vi "LED Control.vi"(11 "All Robot Commands In":T5) -> ()   [LabVIEW 2016]
uses:
  Drive and Climb SS/Drive + Climb Commands 2017.ctl
  Gear Delivery SS/Gear Delivery Commands.ctl
  Conveyor and Shooter SS/Conveyor and Shooter Commands.ctl
  Ball Intake SS/Ball Intake Commands.ctl
  Global Variables/Refnum Names.vi
  Global Variables/Robot Status.vi
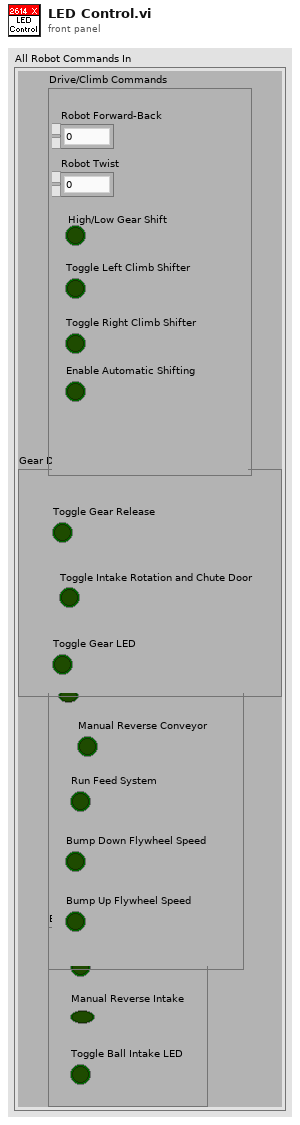
[diagram p1: front panel]
types:
  T1 = typedef "Drive + Climb Commands 2017.ctl" = cluster{"Robot Forward-Back":dbl, "Robot Twist":dbl, "High/Low Gear Shift":bool, "Toggle Left Climb Shifter":bool, "Toggle Right Climb Shifter":bool, "Enable Automatic Shifting":bool}
  T2 = typedef "Gear Delivery Commands.ctl" = cluster{"Toggle Gear Release":bool, "Toggle Intake Rotation and Chute Door":bool, "Toggle Gear LED":bool}
  T3 = typedef "Conveyor and Shooter Commands.ctl" = cluster{"Toggle Shooter":bool, "Manual Reverse Conveyor":bool, "Run Feed System":bool, "Bump Down Flywheel Speed":bool, "Bump Up Flywheel Speed":bool}
  T4 = typedef "Ball Intake Commands.ctl" = cluster{"Toggle Ball Intake":bool, "Manual Reverse Intake":bool, "Toggle Ball Intake LED":bool}
  T5 = cluster{"Drive/Climb Commands":T1, "Gear Delivery Commands":T2, "Shooter and Conveyor Commands":T3, "Ball Intake Commands":T4}
  T6 = typedef "WPI_MotorControlDeviceRef.ctl" = cluster{"DeviceStatus":errorcluster, "Type":T7, "PWM":cluster{"PWM Channel":T8, "DeadBand":T9}, "CAN":cluster{"Device Number":u8, "SetOutput VI Ref":variant, "GetOutput VI Ref":variant, "Enable VI Ref":variant, "Disable VI Ref":variant, "Data":variant}, "Invert":bool}
  T7 = typedef "WPI_MotorControlType.ctl" = enum16{"PWM", "CAN"}
  T8 = typedef "FPGA_DIOPWMChannel.ctl" = enum8{"PWM 0", "PWM 1", "PWM 2", "PWM 3", "PWM 4", "PWM 5", "PWM 6", "PWM 7", "PWM 8", "PWM 9", "PWM MXP 0", "PWM MXP 1", "PWM MXP 2", "PWM MXP 3", "PWM MXP 4", "PWM MXP 5", "PWM MXP 6", "PWM MXP 7", "PWM MXP 8", "PWM MXP 9", "Invalid"}
  T9 = typedef "WPI_PWMDeadband.ctl" = cluster{"Name":string, "maxPositivePwm":i32, "minPositivePwm":i32, "centerPwm":i32, "maxNegativePwm":i32, "minNegativePwm":i32, "angularRange":u16}
  T10 = typedef "WPI_DigitalOutputDevRef.ctl" = cluster{"DIO Channel":T11, "DevStatus":errorcluster}
  T11 = typedef "FPGA_DIOChannel.ctl" = enum8{"DIO 0", "DIO 1", "DIO 2", "DIO 3", "DIO 4", "DIO 5", "DIO 6", "DIO 7", "DIO 8", "DIO 9", "DIO MXP 0", "DIO MXP 1", "DIO MXP 2", "DIO MXP 3", "DIO MXP 4", "DIO MXP 5", "DIO MXP 6", "DIO MXP 7", "DIO MXP 8", "DIO MXP 9", "DIO MXP 10", "DIO MXP 11", "DIO MXP 12", "DIO MXP 13", "DIO MXP 14", "DIO MXP 15", "SPI Port CS1", "SPI Port CS2", "SPI Port CS3", "SPI Port MISO", "SPI Port MOSI", "Invalid"}
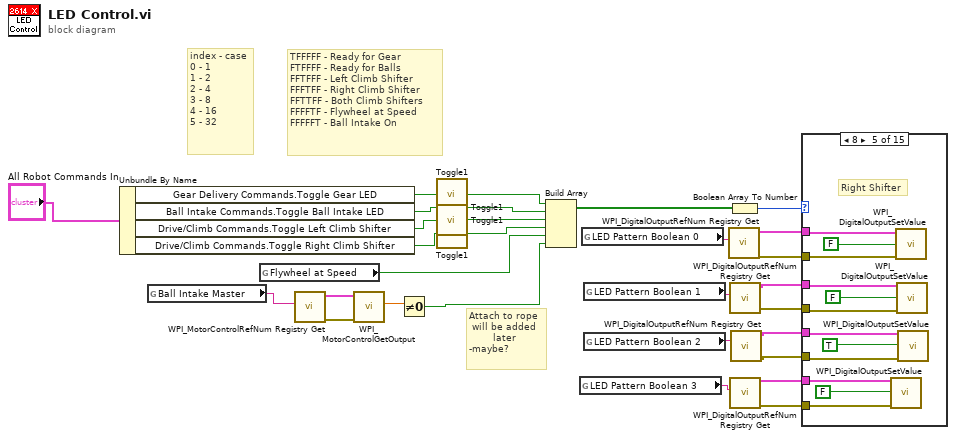
[diagram p0: block diagram]
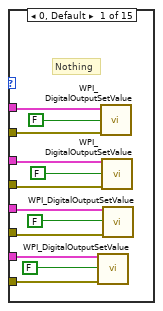
[diagram p2: hidden frame]
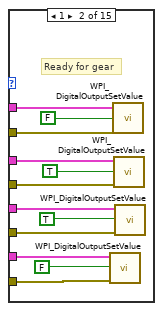
[diagram p3: hidden frame]
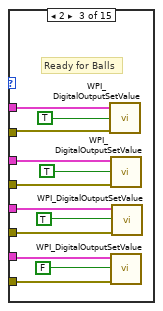
[diagram p4: hidden frame]
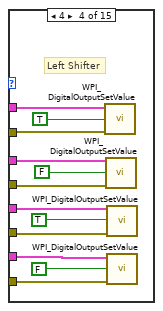
[diagram p5: hidden frame]
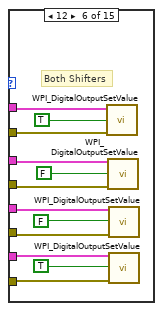
[diagram p6: hidden frame]
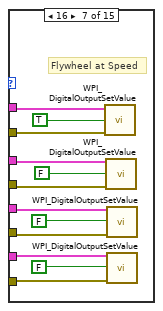
[diagram p7: hidden frame]
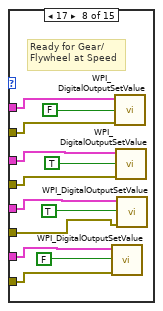
[diagram p8: hidden frame]
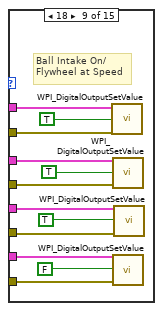
[diagram p9: hidden frame]
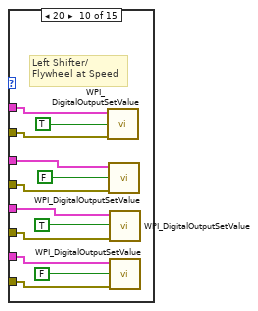
[diagram p10: hidden frame]
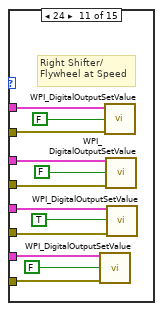
[diagram p11: hidden frame]
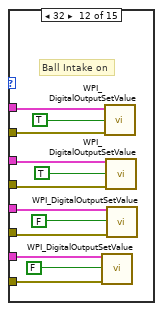
[diagram p12: hidden frame]
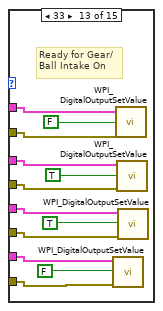
[diagram p13: hidden frame]
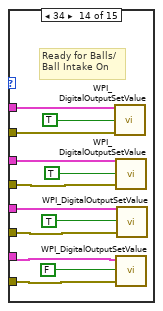
[diagram p14: hidden frame]
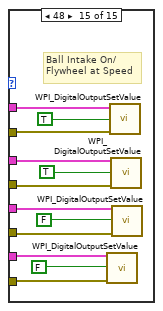
[diagram p15: hidden frame]
diagram:
  # "index - case\n0 - 1\n1 - 2\n2 - 4\n3 - 8\n4 - 16\n5 - 32"
  # "TFFFFF - Ready for Gear\nFTFFFF - Ready for Balls\nFFTFFF - Left Climb Shifter\nFFFTFF - Right Climb Shifter\nFFTTFF - Both Climb Shifters\nFFFFTF - Flywheel at Speed\nFFFFFT - Ball Intake On"
  # "Attach to rope\n will be added \n        later\n-maybe?"
  n1 = Unbundle By Name("All Robot Commands In") -> ("Gear Delivery Commands.Toggle Gear LED"=w11:bool, "Ball Intake Commands.Toggle Ball Intake LED"=w9:bool, "Drive/Climb Commands.Toggle Left Climb Shifter"=w15:bool, "Drive/Climb Commands.Toggle Right Climb Shifter"=w14:bool)
  n2 = global read "Refnum Names.vi" "Ball Intake Master"() -> (w8:string)
  n3 = global read "Robot Status.vi" "Flywheel at Speed"() -> (w4:bool)
  n4 = call <vilib>:"WPI_MotorControlRefNum Registry Get.vi"("refnum name"=w8) -> ("error out"=w7:errorcluster, "MotorControlDevRef"=w6:T6)  [unwired: 9 in]
  n5 = call <vilib>:"WPI_MotorControlGetOutput.vi"("error in"=w7, "MotorControlDevRef"=w6) -> ("Output"=w5:dbl)  [unwired: 7 in, 2 out]
  n6 = Not Equal To 0?(x=w5) -> (x != 0?=w3:bool)
  n7 = call "Toggle1.vi"("Boolean"=w11) -> ("Driver Switch 2"=w1:bool)
  n8 = call "Toggle1.vi"("Boolean"=w9) -> ("Driver Switch 2"=w10:bool)
  n9 = call "Toggle1.vi"("Boolean"=w15) -> ("Driver Switch 2"=w2:bool)
  n10 = call "Toggle1.vi"("Boolean"=w14) -> ("Driver Switch 2"=w12:bool)
  n11 = Build Array(w1, w10, w2, w12, w4, w3) -> (w22:bool[])
  n12 = global read "Refnum Names.vi" "LED Pattern Boolean 3"() -> (w13:string)
  n13 = global read "Refnum Names.vi" "LED Pattern Boolean 0"() -> (w20:string)
  n14 = global read "Refnum Names.vi" "LED Pattern Boolean 1"() -> (w18:string)
  n15 = global read "Refnum Names.vi" "LED Pattern Boolean 2"() -> (w19:string)
  n16 = call <vilib>:"WPI_DigitalOutputRefNum Registry Get.vi"("refnum name"=w20) -> ("error out"=w28:errorcluster, "DigitalOutputDevRef"=w23:T10)  [unwired: 9 in]
  n17 = Boolean Array To Number(Boolean array=w22) -> (number=w21:u32)
  n18 = call <vilib>:"WPI_DigitalOutputRefNum Registry Get.vi"("refnum name"=w18) -> ("error out"=w26:errorcluster, "DigitalOutputDevRef"=w27:T10)  [unwired: 9 in]
  n19 = call <vilib>:"WPI_DigitalOutputRefNum Registry Get.vi"("refnum name"=w13) -> ("error out"=w16:errorcluster, "DigitalOutputDevRef"=w17:T10)  [unwired: 9 in]
  n20 = call <vilib>:"WPI_DigitalOutputRefNum Registry Get.vi"("refnum name"=w19) -> ("error out"=w24:errorcluster, "DigitalOutputDevRef"=w25:T10)  [unwired: 9 in]
  n21 = case shown="8" w21 {
    tunnel: w23 -> [w38 w50 w62 w74 w86 w99 w110 w121 w133 w145 w158 w170 w181 w193 w205]
    tunnel: w28 -> [w37 w49 w61 w73 w85 w98 w109 w120 w132 w144 w157 w169 w180 w192 w204]
    tunnel: w27 -> [w36 w48 w60 w72 w84 w97 w108 w119 w131 w143 w156 w168 w179 w191 w203]
    tunnel: w26 -> [w35 w47 w59 w71 w83 w96 w107 w118 w130 w142 w155 w167 w178 w190 w202]
    tunnel: w25 -> [w34 w46 w58 w70 w82 w95 w106 w117 w129 w141 w154 w166 w177 w189 w201]
    tunnel: w24 -> [w33 w45 w57 w69 w81 w94 w105 w116 w128 w140 w153 w165 w176 w188 w200]
    tunnel: w17 -> [w32 w43 w55 w67 w79 w93 w104 w115 w127 w139 w152 w163 w175 w187 w199]
    tunnel: w16 -> [w30 w42 w54 w66 w78 w92 w103 w114 w126 w138 w151 w162 w174 w186 w198]
    frame 0, Default {
      # "Nothing"
      n22 = call <vilib>:"WPI_DigitalOutputSetValue.vi"("error in (no error)"=w30, "Value"=FALSE, "DigitalOutputDevRef"=w32) -> ()  [unwired: 7 in, 2 out]
      n23 = call <vilib>:"WPI_DigitalOutputSetValue.vi"("error in (no error)"=w37, "Value"=FALSE, "DigitalOutputDevRef"=w38) -> ()  [unwired: 7 in, 2 out]
      n24 = call <vilib>:"WPI_DigitalOutputSetValue.vi"("error in (no error)"=w35, "Value"=FALSE, "DigitalOutputDevRef"=w36) -> ()  [unwired: 7 in, 2 out]
      n25 = call <vilib>:"WPI_DigitalOutputSetValue.vi"("error in (no error)"=w33, "Value"=FALSE, "DigitalOutputDevRef"=w34) -> ()  [unwired: 7 in, 2 out]
    }
    frame 1 {
      # "Ready for gear"
      n26 = call <vilib>:"WPI_DigitalOutputSetValue.vi"("error in (no error)"=w42, "Value"=FALSE, "DigitalOutputDevRef"=w43) -> ()  [unwired: 7 in, 2 out]
      n27 = call <vilib>:"WPI_DigitalOutputSetValue.vi"("error in (no error)"=w49, "Value"=FALSE, "DigitalOutputDevRef"=w50) -> ()  [unwired: 7 in, 2 out]
      n28 = call <vilib>:"WPI_DigitalOutputSetValue.vi"("error in (no error)"=w47, "Value"=TRUE, "DigitalOutputDevRef"=w48) -> ()  [unwired: 7 in, 2 out]
      n29 = call <vilib>:"WPI_DigitalOutputSetValue.vi"("error in (no error)"=w45, "Value"=TRUE, "DigitalOutputDevRef"=w46) -> ()  [unwired: 7 in, 2 out]
    }
    frame 2 {
      # "Ready for Balls"
      n30 = call <vilib>:"WPI_DigitalOutputSetValue.vi"("error in (no error)"=w61, "Value"=TRUE, "DigitalOutputDevRef"=w62) -> ()  [unwired: 7 in, 2 out]
      n31 = call <vilib>:"WPI_DigitalOutputSetValue.vi"("error in (no error)"=w59, "Value"=TRUE, "DigitalOutputDevRef"=w60) -> ()  [unwired: 7 in, 2 out]
      n32 = call <vilib>:"WPI_DigitalOutputSetValue.vi"("error in (no error)"=w54, "Value"=FALSE, "DigitalOutputDevRef"=w55) -> ()  [unwired: 7 in, 2 out]
      n33 = call <vilib>:"WPI_DigitalOutputSetValue.vi"("error in (no error)"=w57, "Value"=TRUE, "DigitalOutputDevRef"=w58) -> ()  [unwired: 7 in, 2 out]
    }
    frame 4 {
      # "Left Shifter"
      n34 = call <vilib>:"WPI_DigitalOutputSetValue.vi"("error in (no error)"=w73, "Value"=TRUE, "DigitalOutputDevRef"=w74) -> ()  [unwired: 7 in, 2 out]
      n35 = call <vilib>:"WPI_DigitalOutputSetValue.vi"("error in (no error)"=w71, "Value"=FALSE, "DigitalOutputDevRef"=w72) -> ()  [unwired: 7 in, 2 out]
      n36 = call <vilib>:"WPI_DigitalOutputSetValue.vi"("error in (no error)"=w69, "Value"=TRUE, "DigitalOutputDevRef"=w70) -> ()  [unwired: 7 in, 2 out]
      n37 = call <vilib>:"WPI_DigitalOutputSetValue.vi"("error in (no error)"=w66, "Value"=FALSE, "DigitalOutputDevRef"=w67) -> ()  [unwired: 7 in, 2 out]
    }
    frame 8 {
      # "Right Shifter"
      n38 = call <vilib>:"WPI_DigitalOutputSetValue.vi"("error in (no error)"=w78, "Value"=FALSE, "DigitalOutputDevRef"=w79) -> ()  [unwired: 7 in, 2 out]
      n39 = call <vilib>:"WPI_DigitalOutputSetValue.vi"("error in (no error)"=w85, "Value"=FALSE, "DigitalOutputDevRef"=w86) -> ()  [unwired: 7 in, 2 out]
      n40 = call <vilib>:"WPI_DigitalOutputSetValue.vi"("error in (no error)"=w83, "Value"=FALSE, "DigitalOutputDevRef"=w84) -> ()  [unwired: 7 in, 2 out]
      n41 = call <vilib>:"WPI_DigitalOutputSetValue.vi"("error in (no error)"=w81, "Value"=TRUE, "DigitalOutputDevRef"=w82) -> ()  [unwired: 7 in, 2 out]
    }
    frame 12 {
      # "Both Shifters"
      n42 = call <vilib>:"WPI_DigitalOutputSetValue.vi"("error in (no error)"=w98, "Value"=TRUE, "DigitalOutputDevRef"=w99) -> ()  [unwired: 7 in, 2 out]
      n43 = call <vilib>:"WPI_DigitalOutputSetValue.vi"("error in (no error)"=w96, "Value"=FALSE, "DigitalOutputDevRef"=w97) -> ()  [unwired: 7 in, 2 out]
      n44 = call <vilib>:"WPI_DigitalOutputSetValue.vi"("error in (no error)"=w94, "Value"=FALSE, "DigitalOutputDevRef"=w95) -> ()  [unwired: 7 in, 2 out]
      n45 = call <vilib>:"WPI_DigitalOutputSetValue.vi"("error in (no error)"=w92, "Value"=TRUE, "DigitalOutputDevRef"=w93) -> ()  [unwired: 7 in, 2 out]
    }
    frame 16 {
      # "Flywheel at Speed"
      n46 = call <vilib>:"WPI_DigitalOutputSetValue.vi"("error in (no error)"=w109, "Value"=TRUE, "DigitalOutputDevRef"=w110) -> ()  [unwired: 7 in, 2 out]
      n47 = call <vilib>:"WPI_DigitalOutputSetValue.vi"("error in (no error)"=w107, "Value"=FALSE, "DigitalOutputDevRef"=w108) -> ()  [unwired: 7 in, 2 out]
      n48 = call <vilib>:"WPI_DigitalOutputSetValue.vi"("error in (no error)"=w105, "Value"=FALSE, "DigitalOutputDevRef"=w106) -> ()  [unwired: 7 in, 2 out]
      n49 = call <vilib>:"WPI_DigitalOutputSetValue.vi"("error in (no error)"=w103, "Value"=FALSE, "DigitalOutputDevRef"=w104) -> ()  [unwired: 7 in, 2 out]
    }
    frame 17 {
      # "Ready for Gear/\nFlywheel at Speed"
      n50 = call <vilib>:"WPI_DigitalOutputSetValue.vi"("error in (no error)"=w114, "Value"=FALSE, "DigitalOutputDevRef"=w115) -> ()  [unwired: 7 in, 2 out]
      n51 = call <vilib>:"WPI_DigitalOutputSetValue.vi"("error in (no error)"=w120, "Value"=FALSE, "DigitalOutputDevRef"=w121) -> ()  [unwired: 7 in, 2 out]
      n52 = call <vilib>:"WPI_DigitalOutputSetValue.vi"("error in (no error)"=w118, "Value"=TRUE, "DigitalOutputDevRef"=w119) -> ()  [unwired: 7 in, 2 out]
      n53 = call <vilib>:"WPI_DigitalOutputSetValue.vi"("error in (no error)"=w116, "Value"=TRUE, "DigitalOutputDevRef"=w117) -> ()  [unwired: 7 in, 2 out]
    }
    frame 18 {
      # "Ball Intake On/\nFlywheel at Speed"
      n54 = call <vilib>:"WPI_DigitalOutputSetValue.vi"("error in (no error)"=w132, "Value"=TRUE, "DigitalOutputDevRef"=w133) -> ()  [unwired: 7 in, 2 out]
      n55 = call <vilib>:"WPI_DigitalOutputSetValue.vi"("error in (no error)"=w130, "Value"=TRUE, "DigitalOutputDevRef"=w131) -> ()  [unwired: 7 in, 2 out]
      n56 = call <vilib>:"WPI_DigitalOutputSetValue.vi"("error in (no error)"=w126, "Value"=FALSE, "DigitalOutputDevRef"=w127) -> ()  [unwired: 7 in, 2 out]
      n57 = call <vilib>:"WPI_DigitalOutputSetValue.vi"("error in (no error)"=w128, "Value"=TRUE, "DigitalOutputDevRef"=w129) -> ()  [unwired: 7 in, 2 out]
    }
    frame 20 {
      # "Left Shifter/\nFlywheel at Speed"
      n58 = call <vilib>:"WPI_DigitalOutputSetValue.vi"("error in (no error)"=w144, "Value"=TRUE, "DigitalOutputDevRef"=w145) -> ()  [unwired: 7 in, 2 out]
      n59 = call <vilib>:"WPI_DigitalOutputSetValue.vi"("error in (no error)"=w142, "Value"=FALSE, "DigitalOutputDevRef"=w143) -> ()  [unwired: 7 in, 2 out]
      n60 = call <vilib>:"WPI_DigitalOutputSetValue.vi"("error in (no error)"=w140, "Value"=TRUE, "DigitalOutputDevRef"=w141) -> ()  [unwired: 7 in, 2 out]
      n61 = call <vilib>:"WPI_DigitalOutputSetValue.vi"("error in (no error)"=w138, "Value"=FALSE, "DigitalOutputDevRef"=w139) -> ()  [unwired: 7 in, 2 out]
    }
    frame 24 {
      # "Right Shifter/\nFlywheel at Speed"
      n62 = call <vilib>:"WPI_DigitalOutputSetValue.vi"("error in (no error)"=w151, "Value"=FALSE, "DigitalOutputDevRef"=w152) -> ()  [unwired: 7 in, 2 out]
      n63 = call <vilib>:"WPI_DigitalOutputSetValue.vi"("error in (no error)"=w157, "Value"=FALSE, "DigitalOutputDevRef"=w158) -> ()  [unwired: 7 in, 2 out]
      n64 = call <vilib>:"WPI_DigitalOutputSetValue.vi"("error in (no error)"=w155, "Value"=FALSE, "DigitalOutputDevRef"=w156) -> ()  [unwired: 7 in, 2 out]
      n65 = call <vilib>:"WPI_DigitalOutputSetValue.vi"("error in (no error)"=w153, "Value"=TRUE, "DigitalOutputDevRef"=w154) -> ()  [unwired: 7 in, 2 out]
    }
    frame 32 {
      # "Ball Intake on"
      n66 = call <vilib>:"WPI_DigitalOutputSetValue.vi"("error in (no error)"=w162, "Value"=FALSE, "DigitalOutputDevRef"=w163) -> ()  [unwired: 7 in, 2 out]
      n67 = call <vilib>:"WPI_DigitalOutputSetValue.vi"("error in (no error)"=w169, "Value"=TRUE, "DigitalOutputDevRef"=w170) -> ()  [unwired: 7 in, 2 out]
      n68 = call <vilib>:"WPI_DigitalOutputSetValue.vi"("error in (no error)"=w167, "Value"=TRUE, "DigitalOutputDevRef"=w168) -> ()  [unwired: 7 in, 2 out]
      n69 = call <vilib>:"WPI_DigitalOutputSetValue.vi"("error in (no error)"=w165, "Value"=FALSE, "DigitalOutputDevRef"=w166) -> ()  [unwired: 7 in, 2 out]
    }
    frame 33 {
      # "Ready for Gear/\nBall Intake On"
      n70 = call <vilib>:"WPI_DigitalOutputSetValue.vi"("error in (no error)"=w174, "Value"=FALSE, "DigitalOutputDevRef"=w175) -> ()  [unwired: 7 in, 2 out]
      n71 = call <vilib>:"WPI_DigitalOutputSetValue.vi"("error in (no error)"=w180, "Value"=FALSE, "DigitalOutputDevRef"=w181) -> ()  [unwired: 7 in, 2 out]
      n72 = call <vilib>:"WPI_DigitalOutputSetValue.vi"("error in (no error)"=w178, "Value"=TRUE, "DigitalOutputDevRef"=w179) -> ()  [unwired: 7 in, 2 out]
      n73 = call <vilib>:"WPI_DigitalOutputSetValue.vi"("error in (no error)"=w176, "Value"=TRUE, "DigitalOutputDevRef"=w177) -> ()  [unwired: 7 in, 2 out]
    }
    frame 34 {
      # "Ready for Balls/\nBall Intake On"
      n74 = call <vilib>:"WPI_DigitalOutputSetValue.vi"("error in (no error)"=w192, "Value"=TRUE, "DigitalOutputDevRef"=w193) -> ()  [unwired: 7 in, 2 out]
      n75 = call <vilib>:"WPI_DigitalOutputSetValue.vi"("error in (no error)"=w190, "Value"=TRUE, "DigitalOutputDevRef"=w191) -> ()  [unwired: 7 in, 2 out]
      n76 = call <vilib>:"WPI_DigitalOutputSetValue.vi"("error in (no error)"=w186, "Value"=FALSE, "DigitalOutputDevRef"=w187) -> ()  [unwired: 7 in, 2 out]
      n77 = call <vilib>:"WPI_DigitalOutputSetValue.vi"("error in (no error)"=w188, "Value"=TRUE, "DigitalOutputDevRef"=w189) -> ()  [unwired: 7 in, 2 out]
    }
    frame 48 {
      # "Ball Intake On/\nFlywheel at Speed"
      n78 = call <vilib>:"WPI_DigitalOutputSetValue.vi"("error in (no error)"=w198, "Value"=FALSE, "DigitalOutputDevRef"=w199) -> ()  [unwired: 7 in, 2 out]
      n79 = call <vilib>:"WPI_DigitalOutputSetValue.vi"("error in (no error)"=w204, "Value"=TRUE, "DigitalOutputDevRef"=w205) -> ()  [unwired: 7 in, 2 out]
      n80 = call <vilib>:"WPI_DigitalOutputSetValue.vi"("error in (no error)"=w202, "Value"=TRUE, "DigitalOutputDevRef"=w203) -> ()  [unwired: 7 in, 2 out]
      n81 = call <vilib>:"WPI_DigitalOutputSetValue.vi"("error in (no error)"=w200, "Value"=FALSE, "DigitalOutputDevRef"=w201) -> ()  [unwired: 7 in, 2 out]
    }
  }
